vi "串口发送.vi"(2 "错误输入（无错误）":errorcluster, 3 "Cluster":cluster{"命令":string, "是否写入":bool}={"命令"="*IDN?", "是否写入"=FALSE}, 4 "VISA resource name in":refnum<visa-resource-name>) -> (0 "错误输出":errorcluster, 1 "VISA resource name out":refnum<visa-resource-name>)   [LabVIEW 2019]
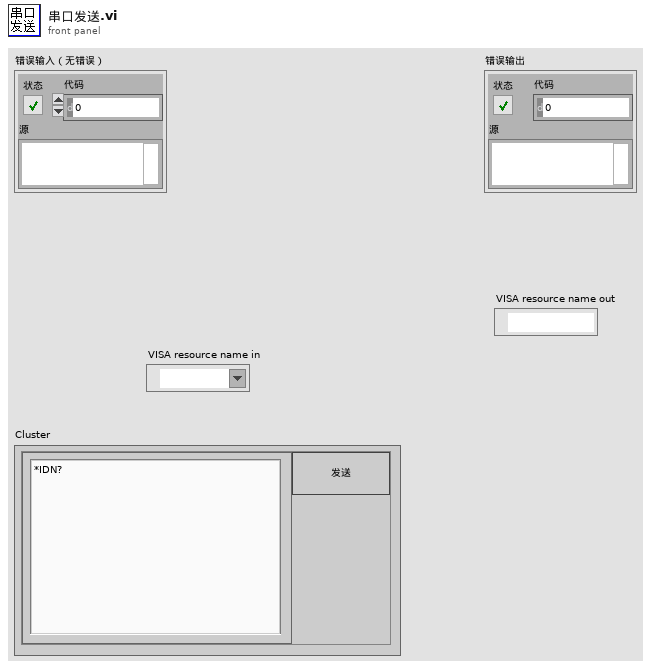
[diagram p1: front panel]
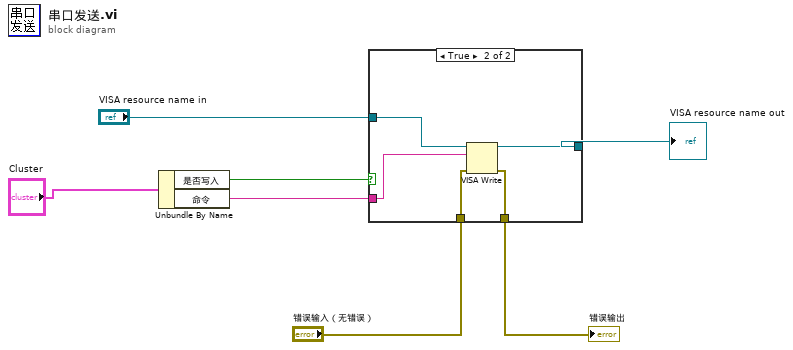
[diagram p0: block diagram]
diagram:
  n1 = Unbundle By Name("Cluster") -> ("是否写入"=w5:bool, "命令"=w7:string)
  n2 = case shown="True" w5 {
    tunnel: "VISA resource name in" -> [w9 w14]
    tunnel: [w9 w13] -> w6
    tunnel: w7 -> [_ w12]
    tunnel: "错误输入（无错误）" -> [w8 w11]
    tunnel: [w8 w10] -> w2
    frame False {
    }
    frame True {
      n3 = VISA Write(VISA resource name=w14, write buffer=w12, error in (no error)=w11) -> (VISA resource name out=w13:refnum<visa-resource-name>, error out=w10:errorcluster)  [unwired: 1 out]
    }
  }
  "VISA resource name out" <- w6
  "错误输出" <- w2
